vi "Status Byte to Code.vi"(8 "error in (no error)":errorcluster, 11 "Status byte [U8]":u8) -> (0 "error out":errorcluster, 3 "Status Code":string)   [LabVIEW 2017, in "Drivers.lvlib" / "ASI TG-1000.lvlib"]
uses:
  ASI TG-1000.lvlib
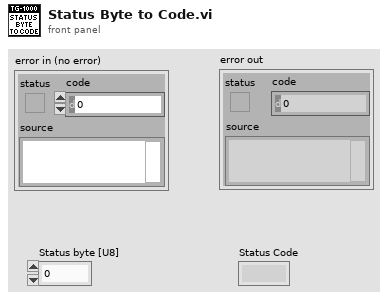
[diagram p1: front panel]
types:
  T1 = cluster{"Boolean array[0]":bool, "Boolean array[1]":bool, "Boolean array[2]":bool, "Boolean array[3]":bool, "Boolean array[4]":bool, "Boolean array[5]":bool, "Boolean array[6]":bool, "Boolean array[7]":bool, "Boolean array[8]":bool}
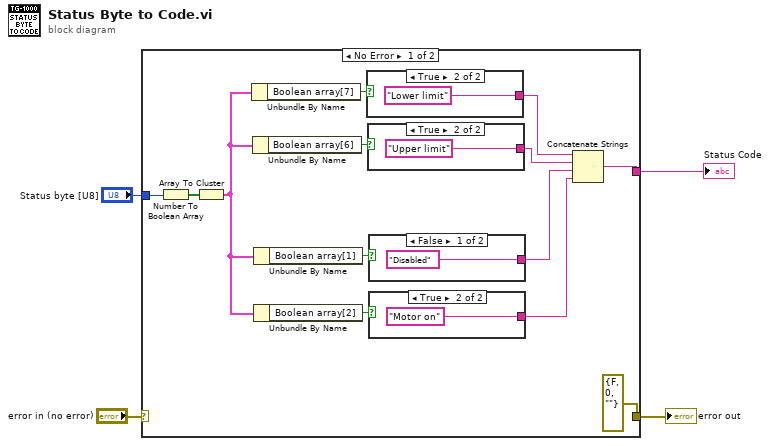
[diagram p0: block diagram]
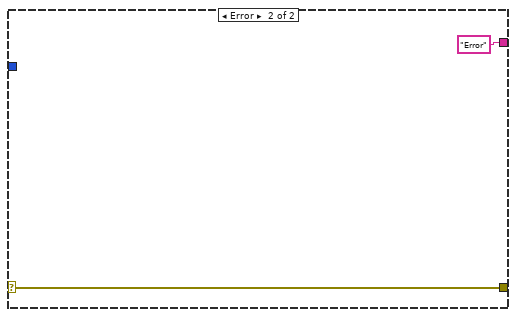
[diagram p6: hidden frame]
diagram:
  n1 = case shown="No Error" "error in (no error)" {
    selector: "error in (no error)" -> [_ w23]
    tunnel: [errorcluster {"status"=FALSE, "code"=0, "source"=""} ("error IO") w23] -> w3
    tunnel: "Status byte [U8]" -> [w17 _]
    tunnel: [w5 "Error"] -> w1
    frame No Error {
      n2 = Number To Boolean Array(number=w17) -> (Boolean array=w16:bool[])
      n3 = Array To Cluster(array=w16) -> (cluster=w10:T1)
      n4 = Unbundle By Name(w10) -> ("Boolean array[7]"=w14:bool)
      n5 = Unbundle By Name(w10) -> ("Boolean array[6]"=w13:bool)
      n6 = Unbundle By Name(w10) -> ("Boolean array[1]"=w12:bool)
      n7 = Unbundle By Name(w10) -> ("Boolean array[2]"=w11:bool)
      n8 = case shown="True" w14 {
        tunnel: [_ "Lower limit"] -> w9
        frame False {
        }
        frame True {
        }
      }
      n9 = case shown="True" w13 {
        tunnel: [_ "Upper limit"] -> w8
        frame False {
        }
        frame True {
        }
      }
      n10 = case shown="False" w12 {
        tunnel: ["Disabled" _] -> w6
        frame False {
        }
        frame True {
        }
      }
      n11 = case shown="True" w11 {
        tunnel: [_ "Motor on"] -> w7
        frame False {
        }
        frame True {
        }
      }
      n12 = Concatenate Strings(w9, w8, w6, w7) -> (w5:string)
    }
    frame Error {
    }
  }
  "error out" <- w3
  "Status Code" <- w1
